vi "Get Nearest and Most Ancestral Classes.vi"(8 "error in (no error)":errorcluster, 10 "Simple Method Name":string, 11 "Input Class Ref":refnum<vi>) -> (0 "error out":errorcluster, 2 "Most Ancestral Class Ref":refnum<vi>, 3 "All Class Refnums":refnum<vi>[](array[refnum]), 5 "Nearest Implementor Class Ref":refnum<vi>)   [LabVIEW 2020, in "Peek Window.lvlib" / "Dynamic Dispatch VI Type.lvclass"]
uses:
  Dynamic Dispatch VI Type.lvclass
  Dynamic Dispatch VI Type.lvclass/Dynamic Dispatch VI Type.ctl
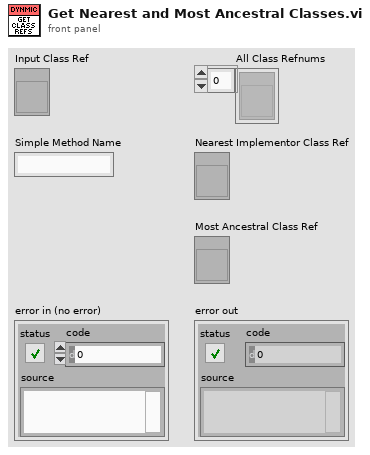
[diagram p1: front panel]
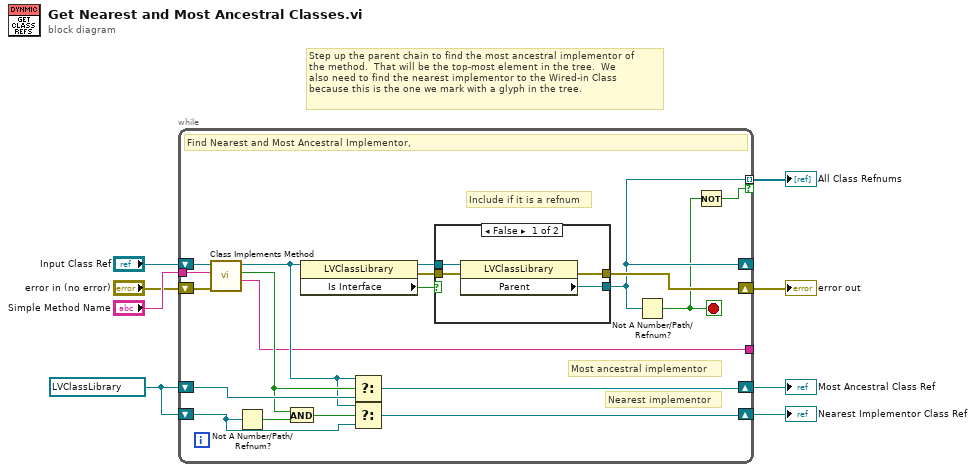
[diagram p0: block diagram]
diagram:
  w2 = refnum<vi> refnum ("Class Refnum out")
  # "Step up the parent chain to find the most ancestral implementor of\nthe method.  That will be the top-most element in the tree.  We\nalso need to find the nearest implementor to the Wired-in Class\nbecause this is the one we mark with a glyph in the tree."
  n1 = while {
    shift-right: [w23] -> w5
    shift-left: w2 -> [w24]
    shift-right: [w11] -> _
    shift-left: "Input Class Ref" -> [w26]
    shift-right: [w17] -> w8
    shift-left: "error in (no error)" -> [w27]
    tunnel: "Simple Method Name" -> [w25]
    shift-right: [w18] -> w1
    shift-left: w2 -> [w19]
    tunnel: [w12] -> _
    tunnel: [w11] -> w4 mode=indexing if=w9
    stop <- w10 stop-if-true
    # "Include if it is a refnum"
    # "Nearest implementor"
    # "Most ancestral implementor"
    # "Find Nearest and Most Ancestral Implementor,"
    n2 = call "Class Implements Method.vi"("error in (no error)"=w27, "Method Name"=w25, "Class Refnum"=w26) -> ("VI Qualified Name"=w12:string, "Implements method?"=w21:bool, "Class Refnum out"=w14:refnum<vi>)  [unwired: 5 in, 1 out]
    n3 = Not A Number/Path/Refnum?(number/path/refnum=w19) -> (NaN/Path/Refnum?=w22:bool)
    n4 = And(x=w21, y=w22) -> (x .and. y?=w20:bool)
    n5 = property class="LVClassLibrary"(reference=w14) -> (reference out=w16:refnum<vi>, error out=w15:errorcluster, "Is Interface"=w13:bool)  [unwired: 1 in]
    n6 = Select(t=w14, s=w21, f=w24) -> (s? t:f=w23:refnum<vi>)
    n7 = Select(t=w14, s=w20, f=w19) -> (s? t:f=w18:refnum<vi>)
    n8 = case shown="False" w13 {
      tunnel: [w31 w32] -> w17
      tunnel: [w30 _] -> w11
      tunnel: w16 -> [w29 _]
      tunnel: w15 -> [w28 w32]
      frame False {
        n9 = property class="LVClassLibrary"(reference=w29, error in=w28) -> (error out=w31:errorcluster, "Parent"=w30:refnum<vi>)  [unwired: 1 out]
      }
      frame True {
      }
    }
    n10 = Not A Number/Path/Refnum?(number/path/refnum=w11) -> (NaN/Path/Refnum?=w10:bool)
    n11 = Not(x=w10) -> (.not. x?=w9:bool)
  }
  "error out" <- w8
  "Most Ancestral Class Ref" <- w5
  "All Class Refnums" <- w4
  "Nearest Implementor Class Ref" <- w1
